vi "prepCI1_tt.vi"   [LabVIEW 2013]
uses:
  <vilib>/DAQmx/create/channels.llb/DAQmx Create Channel (CI-Count Edges).vi
  <vilib>/DAQmx/configure/timing.llb/DAQmx Timing (Sample Clock).vi
  <resource>/objmgr/daqmx.rc
types:
  T1 = typedef "LVRectTypeDef.ctl" = cluster{"Left":i16, "Top":i16, "Right":i16, "Bottom":i16}
  T2 = cluster{"Xpixels":i32, "Vxminref":dbl, "Vxmaxref":dbl, "P":dbl, "Ypixels":i32, "Vyminref":dbl, "Vymaxref":dbl, "srate":sgl, "sAOxy":i32, "timeout":dbl, "type":string, "date":string, "time":string, "Colormap":u16, "Drawing Mode":u16, "Scanning Mode":u16, "square pixels":bool, "square matrix":bool, "Xpixels Img":i32, "Vx-min Img":dbl, "VX-max Img":dbl, "Ypixels Img":i32, "Vy-min Img":dbl, "Vy-max Img ":dbl, "Angle Img":dbl, "autoshutter":bool, "finite":bool, "cont":bool, "wavdet":bool, "measpoints":i32, "avpp":i32, "bufferAO":i32, "bufferAI":i32, "starttick":u32, "waveform":path, "Vx-ref":dbl, "Vy-ref":dbl, "refreshrate":dbl, "refreshbuffer":i32, "tt_cycles":i32, "motorref":refnum<k7>, "mirrorswitch":refnum<k7>, "sample mode":i32, "maxbufferAI":i32, "sampletreshold":dbl, "srateAODO":sgl, "bin":sgl, "Pel":sgl, "Angle draw":dbl, "srate Img":sgl, "ROIimg_plotbounds":T1, "auto OD":bool, "ODfilt":u16, "reset AO_DO":bool, "aAI":i32[], "aCI":i32[], "aAO":i32[], "aDO":i32[]}
  T3 = cluster{"StageS":i32, "StageL":i32, "data dir":path, "image OD":u16, "contour OD":u16, "point OD":u16, "AOlines":tag[], "AIlines":tag[], "CI lines":tag[], "DO lines":tag[], "AO names":string[], "CI names":string[], "AI names":string[], "DO names":string[]}
  T4 = cluster{"CI":refnum<k21>[], "E_CI":errorcluster[]}
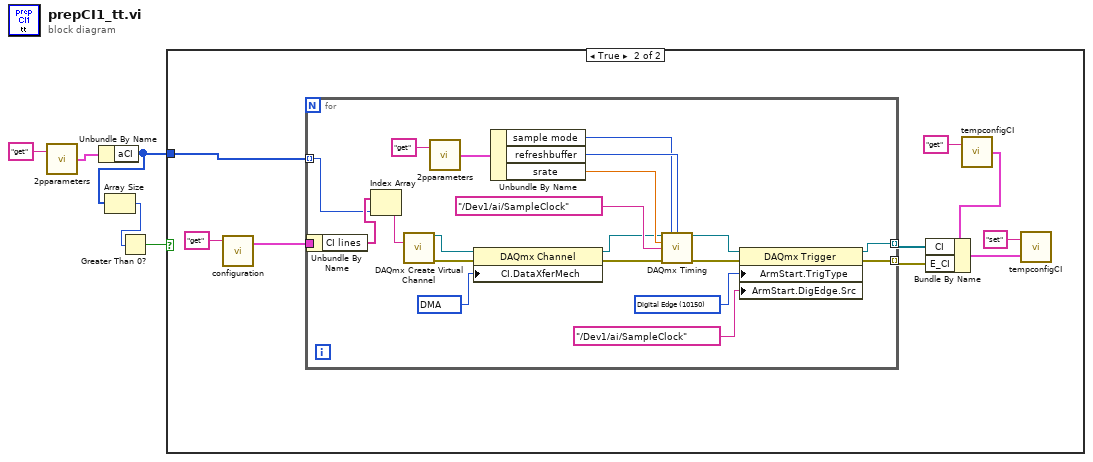
[diagram p0: block diagram]
diagram:
  n1 = call "2pparameters.vi"("command"="get") -> ("params out"=w4:T2)  [unwired: 1 in]
  n2 = Unbundle By Name(w4) -> ("aCI"=w1:i32[])
  n3 = Array Size(array=w1) -> (size(s)=w2:i32)
  n4 = Greater Than 0?(x=w2) -> (x > 0?=w3:bool)
  n5 = case shown="True" w3 {
    tunnel: w1 -> [_ w8]
    frame False {
    }
    frame True {
      n6 = call "configuration.vi"("command"="get") -> ("config out"=w13:T3)  [unwired: 2 in, 1 out]
      n7 = for {
        tunnel: w13 -> [w31]
        tunnel: w8 -> [w18] mode=indexing
        tunnel: [w16] -> w7 mode=indexing
        tunnel: [w15] -> w6 mode=indexing
        w22 = 10054 items=["DMA"=10054, "Interrupts"=10204, "Programmed I/O"=10264, "USB Bulk"=12590] ("CI.DataXferMech")
        w34 = 10150 items=["Digital Edge"=10150, "None"=10230] ("ArmStart.TrigType")
        n8 = Unbundle By Name(w31) -> ("CI lines"=w19:tag[])
        n9 = Index Array(array=w19, index=w18) -> (element=w17:tag)
        n10 = call-poly <vilib>:"DAQmx Create Virtual Channel.vi"("counter"=w17) -> ("task out"=w32:refnum<k21>, "error out"=w21:errorcluster)  [unwired: 13 in]
        n11 = call "2pparameters.vi"("command"="get") -> ("params out"=w28:T2)  [unwired: 1 in]
        n12 = property class="DAQmx Channel"(reference=w32, error in=w21, "CI.DataXferMech"=w22) -> (reference out=w23:refnum<k21>, error out=w20:errorcluster)
        n13 = Unbundle By Name(w28) -> ("sample mode"=w24:i32, "refreshbuffer"=w26:i32, "srate"=w25:sgl)
        n14 = call-poly <vilib>:"DAQmx Timing.vi"("task/channels in"=w23, "sample mode"=w24, "samples per channel"=w26, "rate"=w25, "source"=tag "/Dev1/ai/SampleClock", "error in"=w20) -> ("task out"=w29:refnum<k21>, "error out"=w35:errorcluster)  [unwired: 8 in]
        n15 = property class="DAQmx Trigger"(reference=w29, error in=w35, "ArmStart.TrigType"=w34, "ArmStart.DigEdge.Src"=tag "/Dev1/ai/SampleClock") -> (reference out=w16:refnum<k21>, error out=w15:errorcluster)
      }
      n16 = call "tempconfigCI.vi"("command"="get") -> ("Temp Config out"=w9:T4)  [unwired: 1 in]
      n17 = Bundle By Name(cluster=w9, "CI"=w7, "E_CI"=w6) -> (w12:T4)
      n18 = call "tempconfigCI.vi"("Temp Config in"=w12, "command"="set") -> ()  [unwired: 1 out]
    }
  }
